vi "AutoCoordinator.vi"(3 "Stop":bool, 4 "Start":bool, 5 "MotionPlanningNotifiers":T1, 6 "Steps":T3[](array[typedef])) -> (1 "Claw Open":bool, 2 "IntakeState":T2)   [LabVIEW 2017]
uses:
  TypeDef/AutoStep.ctl
  TypeDef/AutoWaypointType.ctl
  Pathfinder/Pathfinder-LabVIEW/Pathfinder-Lib/VIs/Waypoint.ctl
  Implements/Arm/TypeDefs/ArmTargetPosition.ctl
  Implements/TypeDefs/IntakeState.ctl
  TypeDefs/RobotComponents/MotionPlanningNotifiers.ctl
  PathPlannerSupport/TypeDefs/DrivePlanRequest.ctl
  PathPlannerSupport/TypeDefs/DrivePlanResponse.ctl
  Pathfinder/Pathfinder-LabVIEW/Pathfinder-Lib/VIs/Segment.ctl
  Implements/Arm/TypeDefs/ArmPlanRequest.ctl
  Implements/Arm/TypeDefs/ArmPlanResponse.ctl
  General/MotionProfiling/TypeDefs/TrajectoryPoint.ctl
  <vilib>/Rock Robotics/WPI/ThirdParty/Phoenix-LabVIEW/Motor Controller/Controls/CTRE_Phoenix_MotorControl_TrajectoryPointTimeDur.ctl
  ArgosLib/Signal Processing/TypeDefs/EdgeDetector_Type.ctl
  ArgosLib/ArgosLib.lvlib
  Pathfinder/Pathfinder-LabVIEW/Pathfinder-Lib/Pathfinder.lvlib
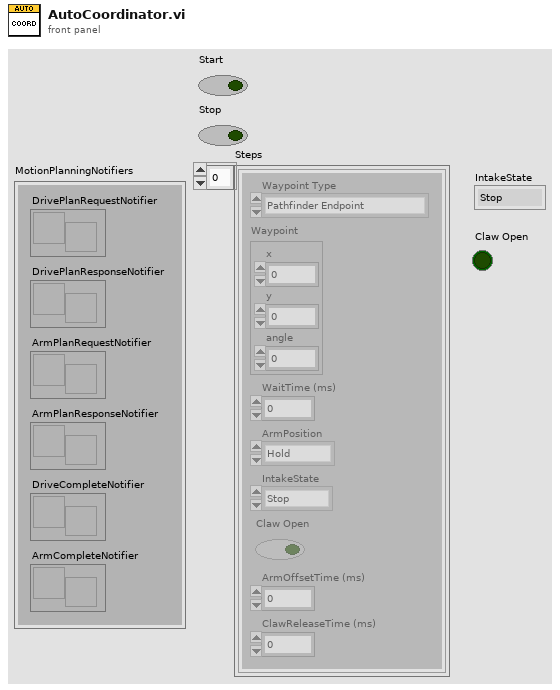
[diagram p1: front panel]
types:
  T1 = typedef "MotionPlanningNotifiers.ctl" = cluster{"DrivePlanRequestNotifier":refnum<notifier>, "DrivePlanResponseNotifier":refnum<notifier>, "ArmPlanRequestNotifier":refnum<notifier>, "ArmPlanResponseNotifier":refnum<notifier>, "DriveCompleteNotifier":refnum<notifier>, "ArmCompleteNotifier":refnum<notifier>}
  T2 = typedef "IntakeState.ctl" = enum16{"Stop", "Forward", "Reverse", "Forward Open"}
  T3 = typedef "AutoStep.ctl" = cluster{"Waypoint Type":T4, "Waypoint":T5, "WaitTime (ms)":u16, "ArmPosition":T6, "IntakeState":T2, "Claw Open":bool, "ArmOffsetTime (ms)":u16, "ClawReleaseTime (ms)":u16}
  T4 = typedef "AutoWaypointType.ctl" = enum16{"Pathfinder Endpoint", "Pathfinder Waypoint", "Zero-Radius Turn Endpoint", "Stationary", "Vision Assist Endpoint", "Stop"}
  T5 = typedef "Pathfinder.lvlib/Waypoint.ctl" = cluster{"x":dbl, "y":dbl, "angle":dbl}
  T6 = typedef "ArmTargetPosition.ctl" = enum16{"Hold", "Switch", "Scale Low", "Scale High", "Climb", "Back Place"}
  T7 = typedef "ArgosLib.lvlib/EdgeDetector_Type.ctl" = enum16{"RisingEdge", "FallingEdge", "Both"}
  T8 = typedef "ArmPlanResponse.ctl" = cluster{"RotateTrajectory":T9[], "ExtendTrajectory":T9[], "PlanTime (ms)":u32, "Execute":bool}
  T9 = typedef "TrajectoryPoint.ctl" = cluster{"Position ":dbl, "Velocity ":dbl, "Time (ms)":T10, "Last Point":bool}
  T10 = typedef "CTRE_Phoenix_MotorControl_TrajectoryPointTimeDur.ctl" = i32
  T11 = typedef "ArmPlanRequest.ctl" = cluster{"Destination":T6, "Preview":bool}
  T12 = typedef "DrivePlanRequest.ctl" = cluster{"Plan Type":T4, "Waypoints":T5[], "Preview":bool}
  T13 = typedef "DrivePlanResponse.ctl" = cluster{"LeftDriveTrajectory":T14[], "RightDriveTrajectory":T14[], "PlanTime (ms)":u32, "Execute":bool}
  T14 = typedef "Pathfinder.lvlib/Segment.ctl" = cluster{"dt":dbl, "x":dbl, "y":dbl, "position":dbl, "velocity":dbl, "acceleration":dbl, "jerk":dbl, "heading":dbl}
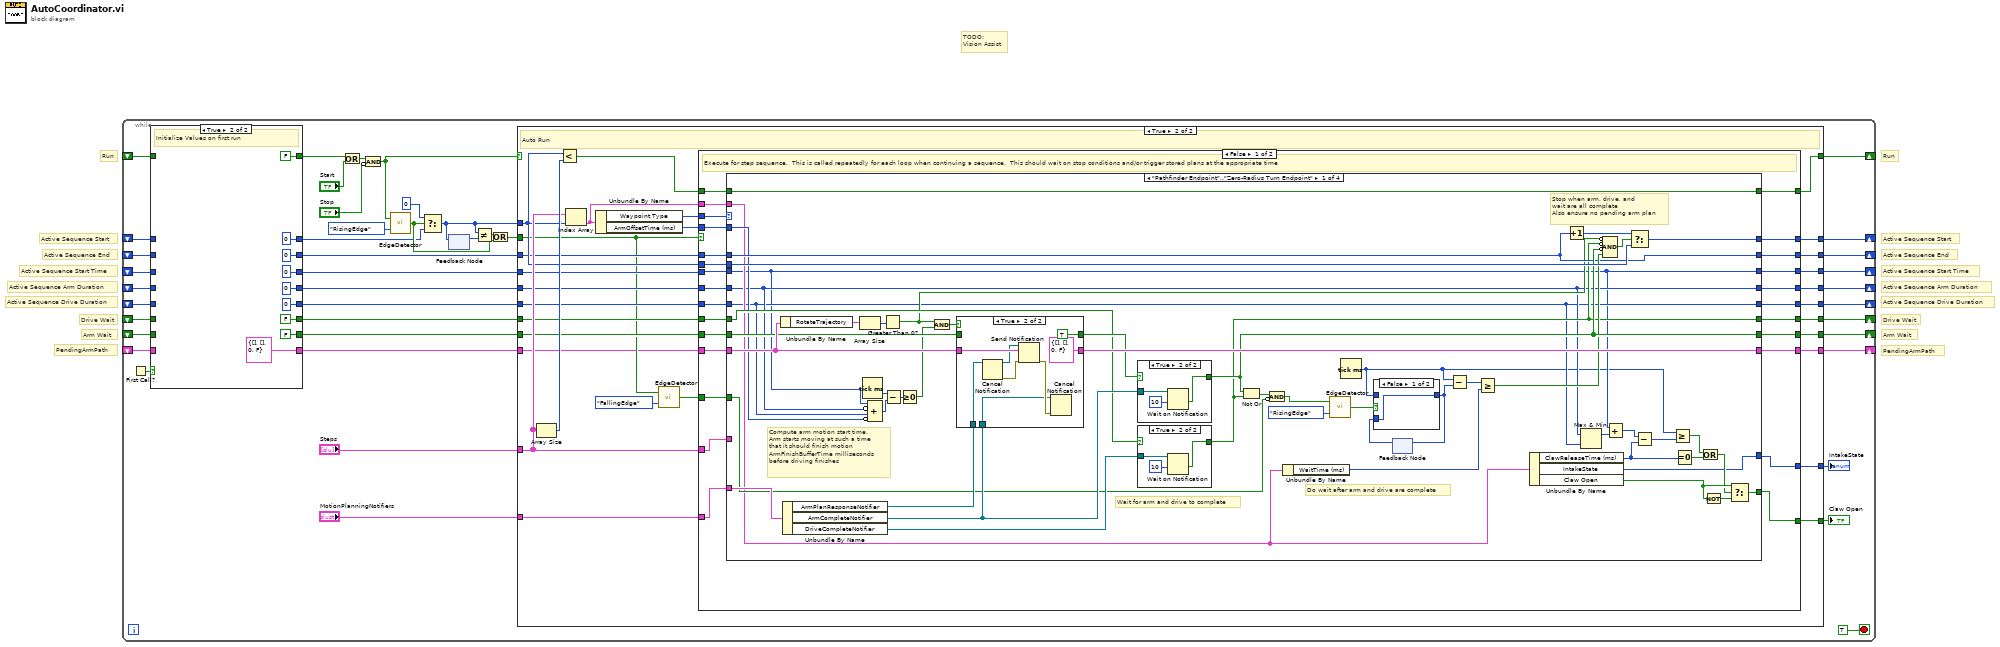
[diagram p0: block diagram]
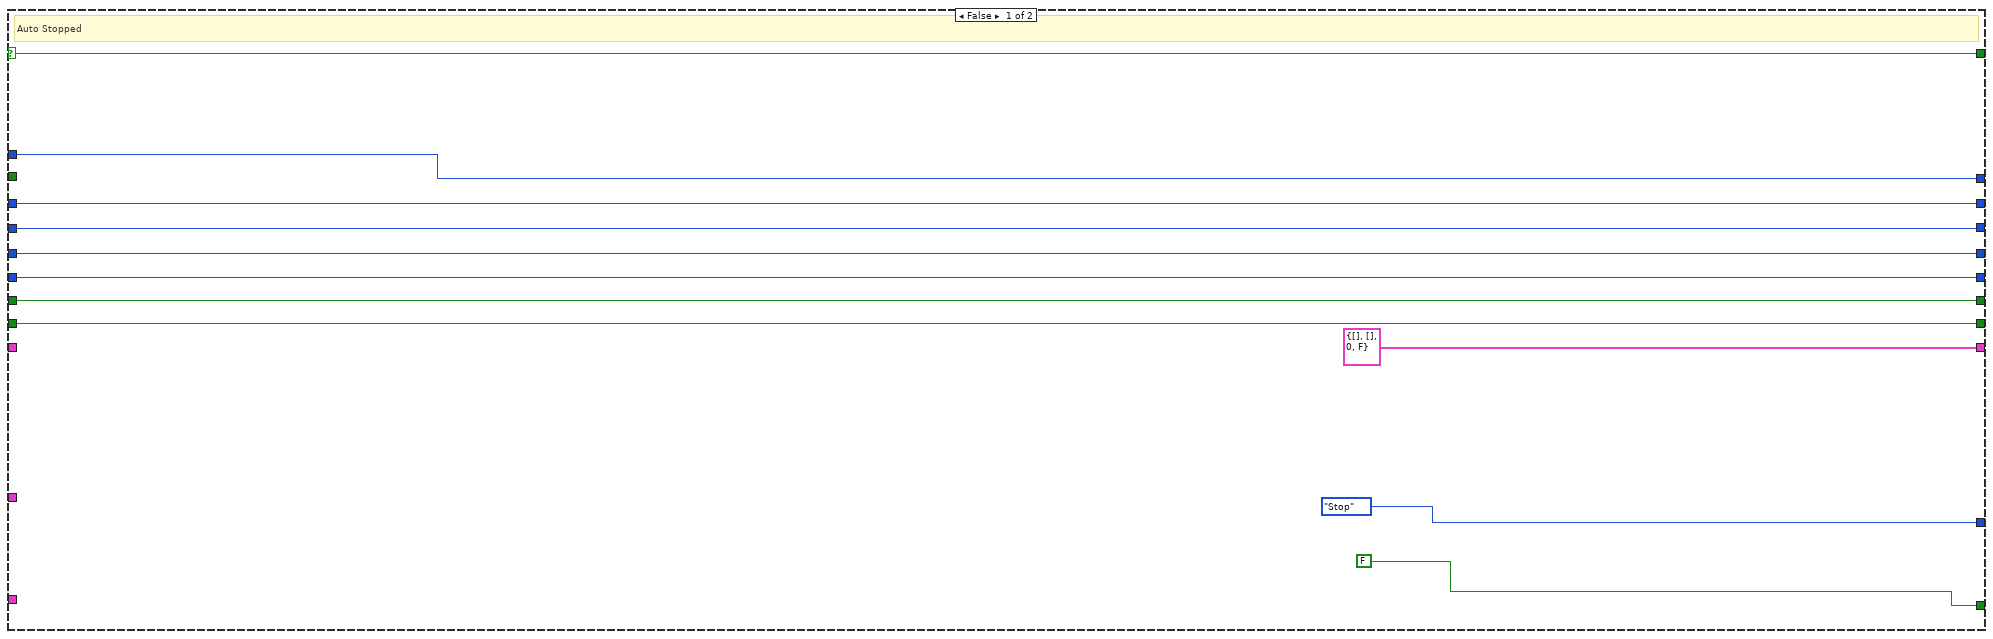
[diagram p3: hidden frame]
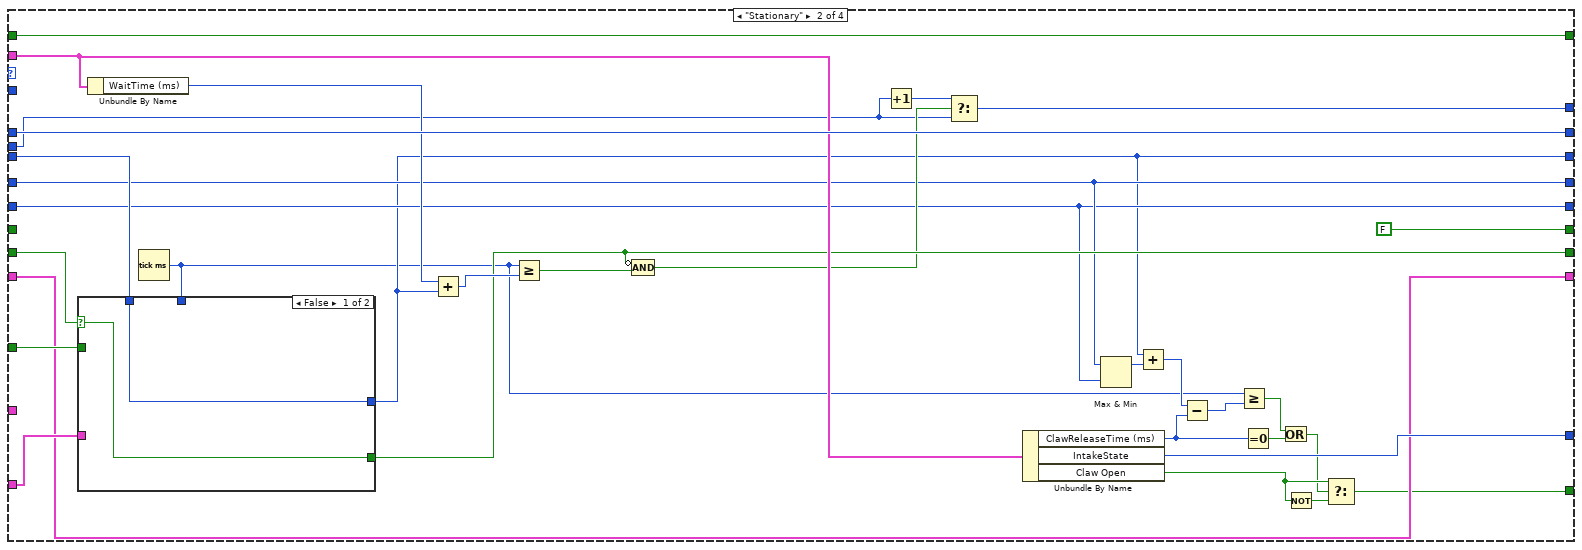
[diagram p8: hidden frame]
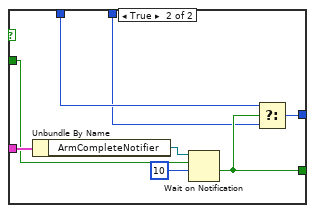
[diagram p9: hidden frame]
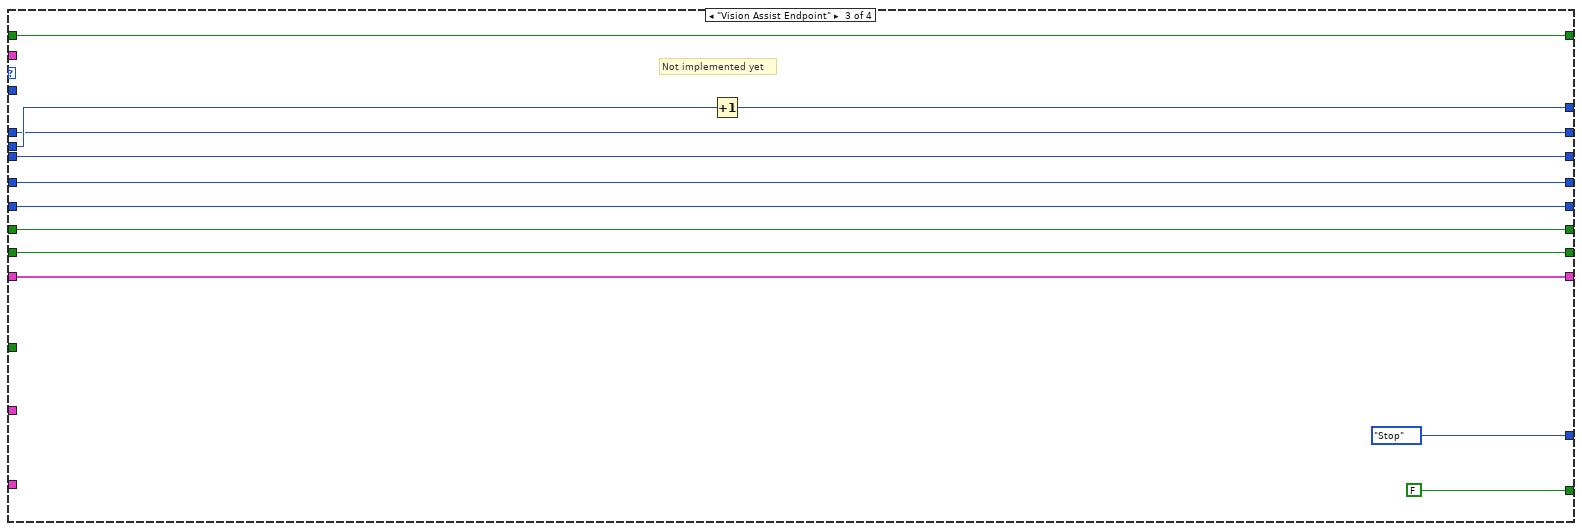
[diagram p10: hidden frame]
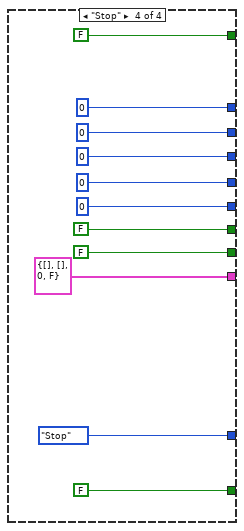
[diagram p11: hidden frame]
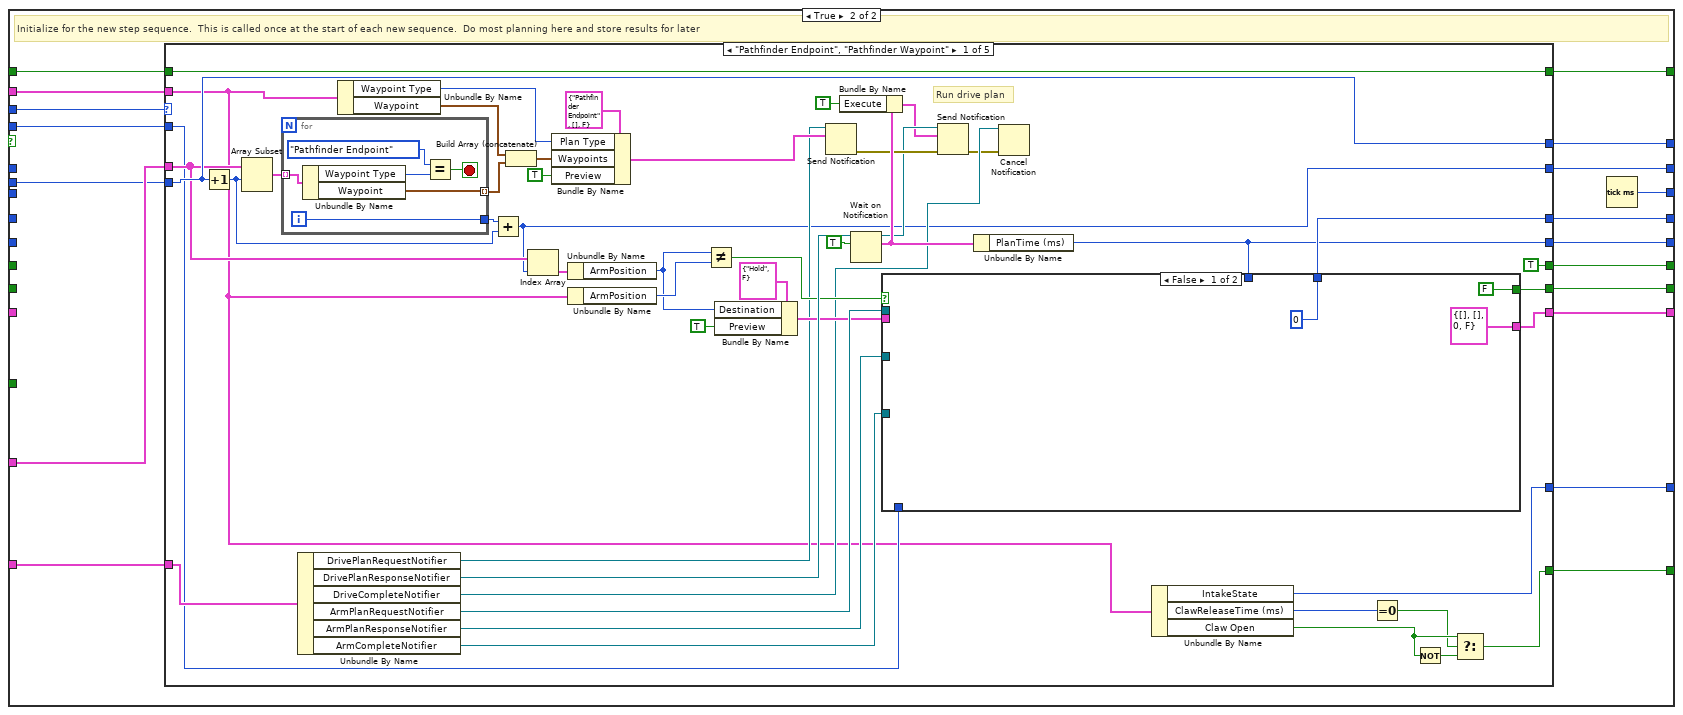
[diagram p12: hidden frame]
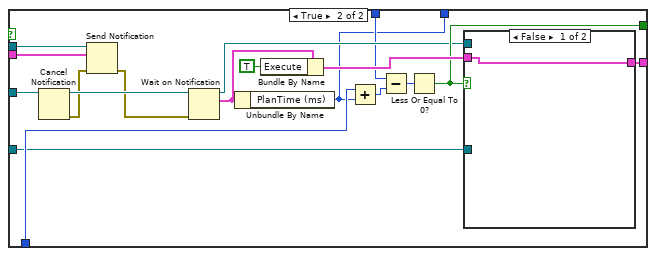
[diagram p13: hidden frame]
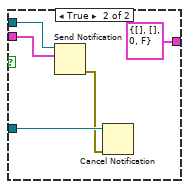
[diagram p14: hidden frame]
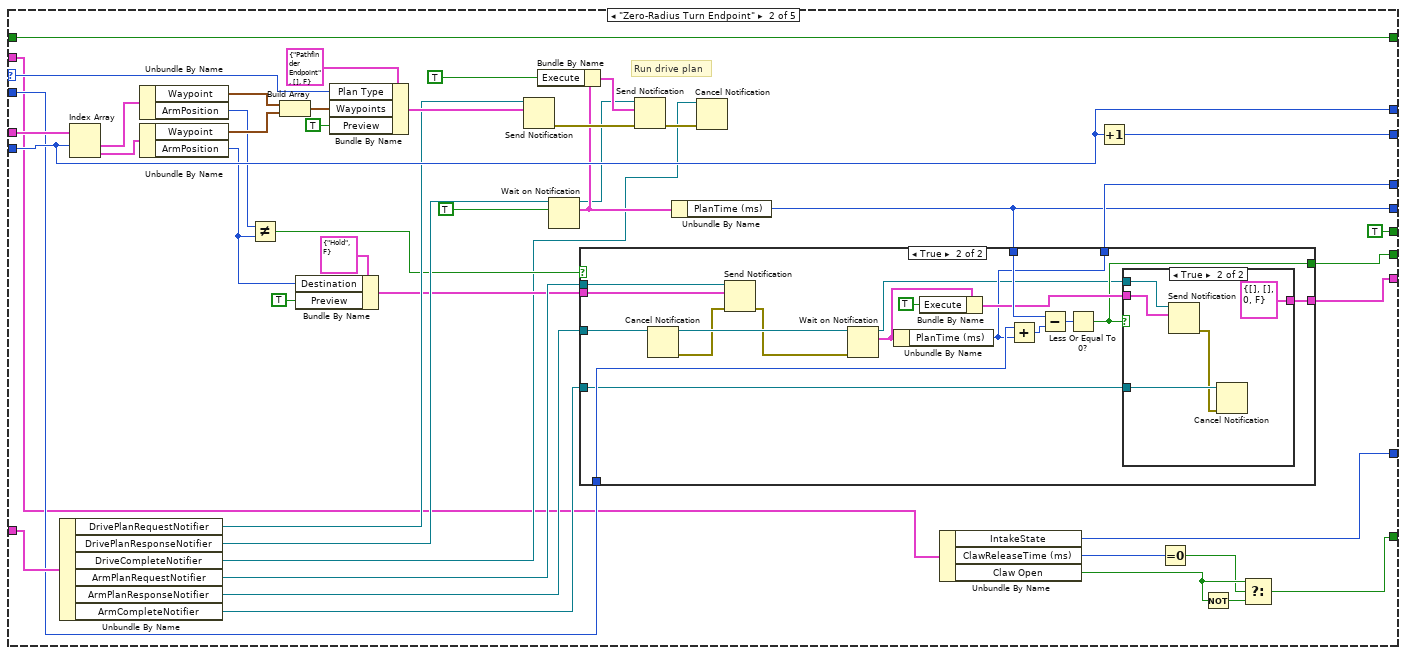
[diagram p15: hidden frame]
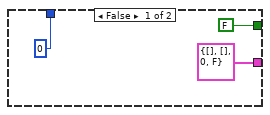
[diagram p16: hidden frame]
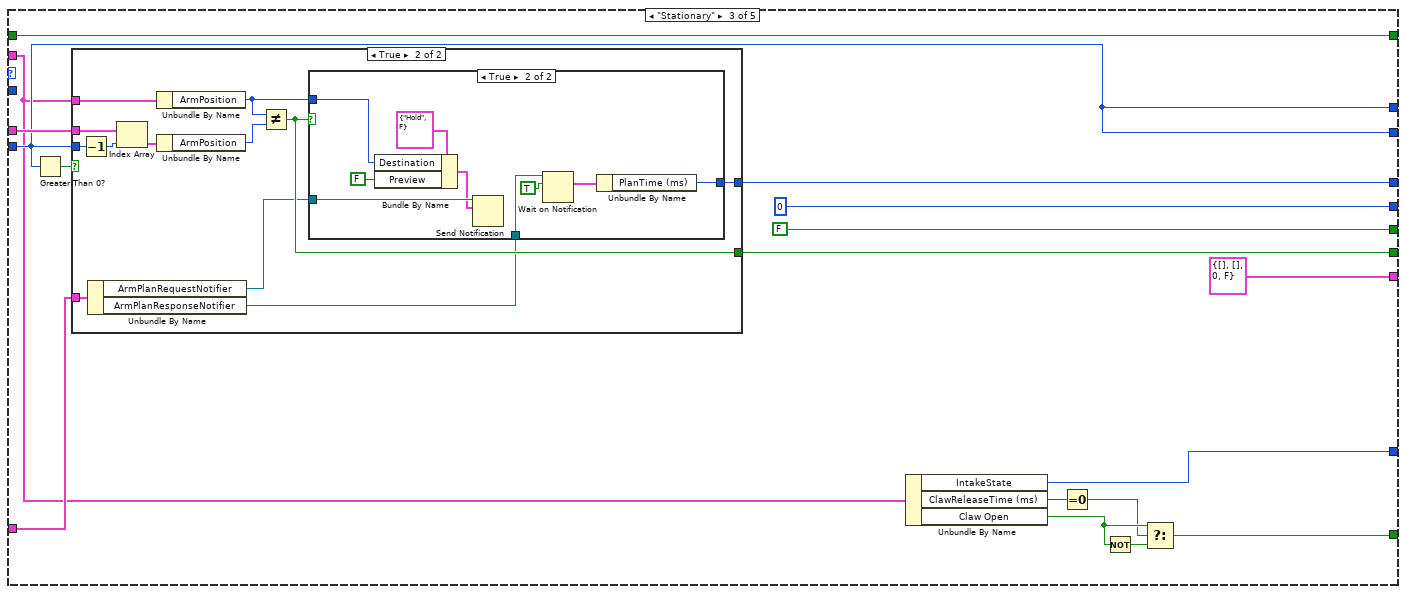
[diagram p18: hidden frame]
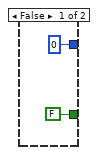
[diagram p19: hidden frame]
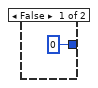
[diagram p20: hidden frame]
diagram:
  # "PendingArmPath"
  # "PendingArmPath"
  # "TODO:\nVision Assist"
  # "Run"
  # "Arm Wait"
  # "Drive Wait"
  # "Active Sequence Drive Duration"
  # "Active Sequence Arm Duration"
  # "Active Sequence Start Time"
  # "Active Sequence End"
  # "Active Sequence Start"
  # "Arm Wait"
  # "Drive Wait"
  # "Active Sequence Drive Duration"
  # "Active Sequence Arm Duration"
  # "Active Sequence Start Time"
  # "Active Sequence End"
  # "Active Sequence Start"
  # "Run"
  n1 = while {
    shift-right: [w37] -> _
    shift-left: _ -> [w17]
    shift-right: [w36] -> _
    shift-left: _ -> [w15]
    shift-right: [w26] -> _
    shift-left: _ -> [w7]
    shift-right: [w25] -> _
    shift-left: _ -> [w6]
    shift-right: [w21] -> _
    shift-left: _ -> [w5]
    shift-right: [w24] -> _
    shift-left: _ -> [w4]
    shift-right: [w23] -> _
    shift-left: _ -> [w3]
    shift-right: [w22] -> _
    shift-left: _ -> [w2]
    shift-right: [w20] -> _
    shift-left: _ -> [w1]
    stop <- TRUE stop-if-true
    n2 = First Call?() -> (First Call?: T/F=w19:bool)
    n3 = case shown="True" w19 {
      tunnel: [w53 FALSE] -> w18
      tunnel: w17 -> [w53 _]
      tunnel: [w52 0] -> w16
      tunnel: w15 -> [w52 _]
      tunnel: [w51 0] -> w14
      tunnel: [w50 u32 0 ("millisecond timer value")] -> w13
      tunnel: [w49 u32 0 ("PlanTime (ms)")] -> w12
      tunnel: [w48 u32 0 ("PlanTime (ms)")] -> w11
      tunnel: [w47 FALSE ("timed out?")] -> w10
      tunnel: [w46 FALSE ("timed out?")] -> w9
      tunnel: [w45 T8 {"RotateTrajectory"=[], "ExtendTrajectory"=[], "PlanTime (ms)"=0, "Execute"=FALSE} ("ArmPlanResponse")] -> w8
      tunnel: w7 -> [w51 _]
      tunnel: w6 -> [w50 _]
      tunnel: w5 -> [w49 _]
      tunnel: w4 -> [w48 _]
      tunnel: w3 -> [w47 _]
      tunnel: w2 -> [w46 _]
      tunnel: w1 -> [w45 _]
      frame False {
      }
      frame True {
        # "Initialize Values on first run"
      }
    }
    n4 = Or(x=w18, y="Start") -> (x .or. y?=w42:bool)
    n5 = Compound Arithmetic op=AND(w42, invert "Stop") -> (w38:bool)
    n6 = call "EdgeDetector.vi"("DetectorType"=EdgeDetector_Type."RisingEdge", "Input"=w38) -> ("Edge"=w28:bool)
    n7 = Select(t=0, s=w28, f=w16) -> (s? t:f=w30:i32)
    n8 = feedback-in #1(w30) -> ()
    n9 = feedback #1() -> (w31:i32)  [unwired: 1 in]
    n10 = Not Equal?(x=w30, y=w31) -> (x != y?=w29:bool)
    n11 = Or(x=w29, y=w28) -> (x .or. y?=w27:bool)
    n12 = case shown="True" w38 {
      selector: w38 -> [w72 _]
      tunnel: [w72 w75] -> w37
      tunnel: w30 -> [w73 w100]
      tunnel: [w73 w99] -> w36
      tunnel: "Steps" -> [_ w101]
      tunnel: [IntakeState."Stop" ("IntakeState") w94] -> w34
      tunnel: [FALSE ("Claw Open") w93] -> w33
      tunnel: "MotionPlanningNotifiers" -> [_ w90]
      tunnel: w27 -> [_ w81]
      tunnel: [w69 w98] -> w26
      tunnel: [w68 w97] -> w25
      tunnel: w13 -> [w68 w96]
      tunnel: [w66 w95] -> w24
      tunnel: [w65 w92] -> w23
      tunnel: [w64 w91] -> w22
      tunnel: [w67 w89] -> w21
      tunnel: w14 -> [w69 w82]
      tunnel: w12 -> [w67 w83]
      tunnel: w11 -> [w66 w84]
      tunnel: w10 -> [w65 w86]
      tunnel: w9 -> [w64 w85]
      tunnel: [T8 {"RotateTrajectory"=[], "ExtendTrajectory"=[], "PlanTime (ms)"=0, "Execute"=FALSE} ("ArmPlanResponse") w78] -> w20
      tunnel: w8 -> [_ w77]
      frame False {
        # "Auto Stopped"
      }
      frame True {
        # "Auto Run"
        n13 = Array Size(array=w101) -> (size(s)=w102:i32)
        n14 = Less?(x=w100, y=w102) -> (x < y?=w76:bool)
        n15 = Index Array(array=w101, index=w100) -> (element=w87:T3)
        n16 = Unbundle By Name(w87) -> ("Waypoint Type"=w88:T4, "ArmOffsetTime (ms)"=w74:u16)
        n17 = call "EdgeDetector.vi"("DetectorType"=EdgeDetector_Type."FallingEdge", "Input"=w81) -> ("Edge"=w79:bool)
        n18 = case shown="False" w81 {
          tunnel: w101 -> [w125 w283]
          tunnel: w100 -> [w119 w282]
          tunnel: [w118 w281] -> w99
          tunnel: [w117 w280] -> w98
          tunnel: [w108 w279] -> w97
          tunnel: w96 -> [w109 _]
          tunnel: [w115 w278] -> w95
          tunnel: [w112 w277] -> w94
          tunnel: [w111 w276] -> w93
          tunnel: [w114 w275] -> w92
          tunnel: [w113 w274] -> w91
          tunnel: w90 -> [w124 w273]
          tunnel: [w116 w272] -> w89
          tunnel: w88 -> [w128 w271]
          tunnel: w87 -> [w126 w270]
          tunnel: w86 -> [w123 _]
          tunnel: w85 -> [w122 _]
          tunnel: w84 -> [w121 _]
          tunnel: w83 -> [w120 _]
          tunnel: w82 -> [w127 _]
          tunnel: w79 -> [w110 _]
          tunnel: [w107 w269] -> w78
          tunnel: w77 -> [w106 _]
          tunnel: w76 -> [w105 w268]
          tunnel: [w104 w267] -> w75
          tunnel: w74 -> [w103 w266]
          frame False {
            # "Execute for step sequence.  This is called repeatedly for each loop when continuing a sequence.  This should wait on stop conditions and/or trigger stored plans at the appropriate time"
            n19 = case shown="\"Pathfinder Endpoint\"..\"Zero-Radius Turn Endpoint\"" w128 {
              tunnel: w127 -> [w151 w227 w248 _]
              tunnel: w126 -> [w133 w226 _ _]
              tunnel: w125 -> [_ _ _ _]
              tunnel: w124 -> [w174 w230 _ _]
              tunnel: w123 -> [w150 _ w252 _]
              tunnel: w122 -> [w170 w232 w251 _]
              tunnel: w121 -> [w131 w208 w253 _]
              tunnel: w120 -> [w132 w209 w254 _]
              tunnel: w109 -> [w130 w225 w245 _]
              tunnel: w119 -> [w178 w217 w250 _]
              tunnel: [w180 w222 w249 0] -> w118
              tunnel: [w151 w227 w248 0] -> w117
              tunnel: [w132 w209 w254 u32 0 ("PlanTime (ms)")] -> w116
              tunnel: [w131 w208 w253 u32 0 ("PlanTime (ms)")] -> w115
              tunnel: [w148 FALSE w252 FALSE ("timed out?")] -> w114
              tunnel: [w162 w220 w251 FALSE ("timed out?")] -> w113
              tunnel: [w134 w231 IntakeState."Stop" ("IntakeState") IntakeState."Stop" ("IntakeState")] -> w112
              tunnel: [w135 w214 FALSE ("Claw Open") FALSE ("Claw Open")] -> w111
              tunnel: w110 -> [w160 w229 _ _]
              tunnel: [w130 w203 w245 u32 0 ("millisecond timer value")] -> w108
              tunnel: [w171 w216 w244 T8 {"RotateTrajectory"=[], "ExtendTrajectory"=[], "PlanTime (ms)"=0, "Execute"=FALSE} ("ArmPlanResponse")] -> w107
              tunnel: w106 -> [w172 w216 w244 _]
              tunnel: w105 -> [w146 w215 w243 _]
              tunnel: [w146 w215 w243 FALSE] -> w104
              tunnel: w103 -> [w145 _ _ _]
              frame "Pathfinder Endpoint".."Zero-Radius Turn Endpoint" {
                # "Do wait after arm and drive are complete"
                # "Wait for arm and drive to complete"
                # "Stop when arm, drive, and\nwait are all complete\nAlso ensure no pending arm plan"
                # "Compute arm motion start time.\nArm starts moving at such a time\nthat it should finish motion\nArmFinishBufferTime milliseconds\nbefore driving finishes"
                n20 = Unbundle By Name(w172) -> ("RotateTrajectory"=w177:T9[])
                n21 = Unbundle By Name(w174) -> ("ArmPlanResponseNotifier"=w173:refnum<notifier>, "ArmCompleteNotifier"=w164:refnum<notifier>, "DriveCompleteNotifier"=w165:refnum<notifier>)
                n22 = Array Size(array=w177) -> (size(s)=w176:i32)
                n23 = Tick Count (ms)() -> (millisecond timer value=w175:u32)
                n24 = Compound Arithmetic op=ADD(w130, invert w132, w131, invert w145) -> (w147:u32)
                n25 = Greater Than 0?(x=w176) -> (x > 0?=w149:bool)
                n26 = Subtract(x=w175, y=w147) -> (x-y=w168:i32)
                n27 = Greater Or Equal To 0?(x=w168) -> (x >= 0?=w167:bool)
                n28 = And(x=w149, y=w167) -> (x .and. y?=w169:bool)
                n29 = case shown="True" w169 {
                  tunnel: [w191 TRUE] -> w163
                  tunnel: w173 -> [_ w195]
                  tunnel: w172 -> [w192 w198]
                  tunnel: w164 -> [_ w197]
                  tunnel: [w192 T8 {"RotateTrajectory"=[], "ExtendTrajectory"=[], "PlanTime (ms)"=0, "Execute"=FALSE} ("ArmPlanResponse")] -> w171
                  tunnel: w170 -> [w191 _]
                  frame False {
                  }
                  frame True {
                    n30 = Cancel Notification(0:w195) -> (8:w194:refnum<notifier>, 11:w193:errorcluster)  [unwired: 1 in, 1 out]
                    n31 = Send Notification(notification=w198, notifier=w194, error in (no error)=w193) -> (error out=w199:errorcluster)  [unwired: 1 out]
                    n32 = Cancel Notification(0:w197, 3:w199) -> ()  [unwired: 3 out]
                  }
                }
                n33 = case shown="True" w163 {
                  selector: w163 -> [w187 _]
                  tunnel: w164 -> [_ w189]
                  tunnel: [w187 w188] -> w162
                  frame False {
                  }
                  frame True {
                    n34 = Wait on Notification(notifier=w189, timeout in ms (-1)=10) -> (timed out?=w188:bool)  [unwired: 2 in, 3 out]
                  }
                }
                n35 = case shown="True" w150 {
                  selector: w150 -> [w183 _]
                  tunnel: w165 -> [_ w185]
                  tunnel: [w183 w184] -> w148
                  frame False {
                  }
                  frame True {
                    n36 = Wait on Notification(notifier=w185, timeout in ms (-1)=10) -> (timed out?=w184:bool)  [unwired: 2 in, 3 out]
                  }
                }
                n37 = Not Or(1:w148, 2:w162) -> (0:w161:bool)
                n38 = Compound Arithmetic op=AND(w161, invert w160) -> (w158:bool)
                n39 = Unbundle By Name(w133) -> ("WaitTime (ms)"=w153:u16)
                n40 = call "EdgeDetector.vi"("DetectorType"=EdgeDetector_Type."RisingEdge", "Input"=w158) -> ("Edge"=w157:bool)
                n41 = Tick Count (ms)() -> (millisecond timer value=w129:u32)
                n42 = feedback #2() -> (w156:u32)  [unwired: 1 in]
                n43 = case shown="False" w157 {
                  tunnel: w129 -> [_ w182]
                  tunnel: [w181 w182] -> w155
                  tunnel: w156 -> [w181 _]
                  frame False {
                  }
                  frame True {
                  }
                }
                n44 = feedback-in #2(w155) -> ()
                n45 = Subtract(x=w129, y=w155) -> (x-y=w154:u32)
                n46 = Greater Or Equal?(x=w154, y=w153) -> (x >= y?=w152:bool)
                n47 = Unbundle By Name(w133) -> ("ClawReleaseTime (ms)"=w140:u16, "IntakeState"=w134:T2, "Claw Open"=w143:bool)
                n48 = Increment(x=w151) -> (x+1=w179:i32)
                n49 = Max & Min(x=w132, y=w131) -> (max(x,y)=w137:u32)  [unwired: 1 out]
                n50 = Compound Arithmetic op=AND(invert w149, invert w148, invert w162, w152) -> (w166:bool)
                n51 = Add(x=w130, y=w137) -> (x+y=w138:u32)
                n52 = Select(t=w179, s=w166, f=w178) -> (s? t:f=w180:i32)
                n53 = Subtract(x=w138, y=w140) -> (x-y=w136:u32)
                n54 = Greater Or Equal?(x=w129, y=w136) -> (x >= y?=w139:bool)
                n55 = Equal To 0?(x=w140) -> (x = 0?=w142:bool)
                n56 = Or(x=w139, y=w142) -> (x .or. y?=w141:bool)
                n57 = Not(x=w143) -> (.not. x?=w144:bool)
                n58 = Select(t=w143, s=w141, f=w144) -> (s? t:f=w135:bool)
              }
              frame "Stationary" {
                n59 = Unbundle By Name(w226) -> ("WaitTime (ms)"=w223:u16)
                n60 = Tick Count (ms)() -> (millisecond timer value=w201:u32)
                n61 = case shown="False" w232 {
                  selector: w232 -> [w234 _]
                  tunnel: w230 -> [_ w242]
                  tunnel: w229 -> [_ w239]
                  tunnel: [w234 w238] -> w220
                  tunnel: w225 -> [w233 w237]
                  tunnel: w201 -> [_ w236]
                  tunnel: [w233 w235] -> w203
                  frame False {
                  }
                  frame True {
                    n62 = Unbundle By Name(w242) -> ("ArmCompleteNotifier"=w241:refnum<notifier>)
                    n63 = Wait on Notification(notifier=w241, ignore previous (F)=w239, timeout in ms (-1)=10) -> (timed out?=w238:bool)  [unwired: 1 in, 3 out]
                    n64 = Select(t=w237, s=w238, f=w236) -> (s? t:f=w235:u32)
                  }
                }
                n65 = Add(x=w223, y=w203) -> (x+y=w224:u32)
                n66 = Greater Or Equal?(x=w201, y=w224) -> (x >= y?=w221:bool)
                n67 = Compound Arithmetic op=AND(invert w220, w221) -> (w219:bool)
                n68 = Increment(x=w217) -> (x+1=w218:i32)
                n69 = Select(t=w218, s=w219, f=w217) -> (s? t:f=w222:i32)
                n70 = Unbundle By Name(w226) -> ("ClawReleaseTime (ms)"=w207:u16, "IntakeState"=w231:T2, "Claw Open"=w212:bool)
                n71 = Max & Min(x=w209, y=w208) -> (max(x,y)=w204:u32)  [unwired: 1 out]
                n72 = Add(x=w203, y=w204) -> (x+y=w205:u32)
                n73 = Subtract(x=w205, y=w207) -> (x-y=w202:u32)
                n74 = Greater Or Equal?(x=w201, y=w202) -> (x >= y?=w206:bool)
                n75 = Equal To 0?(x=w207) -> (x = 0?=w211:bool)
                n76 = Or(x=w206, y=w211) -> (x .or. y?=w210:bool)
                n77 = Not(x=w212) -> (.not. x?=w213:bool)
                n78 = Select(t=w212, s=w210, f=w213) -> (s? t:f=w214:bool)
              }
              frame "Vision Assist Endpoint" {
                # "Not implemented yet"
                n79 = Increment(x=w250) -> (x+1=w249:i32)
              }
              frame "Stop" {
              }
            }
          }
          frame True {
            # "Initialize for the new step sequence.  This is called once at the start of each new sequence.  Do most planning here and store results for later"
            n80 = case shown="\"Pathfinder Endpoint\", \"Pathfinder Waypoint\"" w271 {
              selector: w271 -> [_ w405 _ _ _]
              tunnel: w283 -> [w300 w410 w451 _ _]
              tunnel: w282 -> [w301 w408 w447 w488 _]
              tunnel: w270 -> [w288 w368 w440 _ _]
              tunnel: [w301 w408 w447 w484 0] -> w281
              tunnel: [w299 w409 w447 w484 0] -> w280
              tunnel: [w302 w377 u16 0 u32 0 ("PlanTime (ms)") u32 0 ("PlanTime (ms)")] -> w278
              tunnel: [w284 w365 w439 IntakeState."Stop" ("IntakeState") IntakeState."Stop" ("IntakeState")] -> w277
              tunnel: [w287 w367 w438 FALSE ("Claw Open") FALSE ("Claw Open")] -> w276
              tunnel: [TRUE TRUE FALSE FALSE FALSE] -> w275
              tunnel: [w294 w375 w450 FALSE FALSE] -> w274
              tunnel: w273 -> [w304 w399 w449 _ _]
              tunnel: [w303 w379 w448 u32 0 ("PlanTime (ms)") u32 0 ("PlanTime (ms)")] -> w272
              tunnel: [w295 w380 T8 {"RotateTrajectory"=[], "ExtendTrajectory"=[], "PlanTime (ms)"=0, "Execute"=FALSE} ("ArmPlanResponse") T8 {"RotateTrajectory"=[], "ExtendTrajectory"=[], "PlanTime (ms)"=0, "Execute"=FALSE} ("ArmPlanResponse") T8 {"RotateTrajectory"=[], "ExtendTrajectory"=[], "PlanTime (ms)"=0, "Execute"=FALSE} ("ArmPlanResponse")] -> w269
              tunnel: w268 -> [w292 w373 w445 w479 _]
              tunnel: [w292 w373 w445 w479 FALSE] -> w267
              tunnel: w266 -> [w291 w372 _ _ _]
              frame "Pathfinder Endpoint", "Pathfinder Waypoint" {
                # "Run drive plan"
                n81 = Increment(x=w301) -> (x+1=w329:i32)
                n82 = Array Subset(array=w300, index=w329) -> (w331:T3[])  [unwired: 1 in]
                n83 = for {
                  tunnel: w331 -> [w364] mode=indexing
                  tunnel: [w360] -> w330
                  tunnel: [w359] -> w325 mode=indexing
                  i -> [w360]
                  stop <- w361 stop-if-true
                  n84 = Unbundle By Name(w364) -> ("Waypoint Type"=w363:T4, "Waypoint"=w359:T5)
                  n85 = Equal?(x=AutoWaypointType."Pathfinder Endpoint", y=w363) -> (x = y?=w361:bool)
                }
                n86 = Unbundle By Name(w304) -> ("DrivePlanRequestNotifier"=w305:refnum<notifier>, "DrivePlanResponseNotifier"=w322:refnum<notifier>, "DriveCompleteNotifier"=w312:refnum<notifier>, "ArmPlanRequestNotifier"=w317:refnum<notifier>, "ArmPlanResponseNotifier"=w313:refnum<notifier>, "ArmCompleteNotifier"=w311:refnum<notifier>)
                n87 = Unbundle By Name(w288) -> ("Waypoint Type"=w327:T4, "Waypoint"=w326:T5)
                n88 = Add(x=w330, y=w329) -> (x+y=w299:i32)
                n89 = Build Array (concatenate)(w326, w325) -> (w324:T5[])
                n90 = Index Array(array=w300, index=w299) -> (element=w298:T3)
                n91 = Bundle By Name(cluster=T12 {"Plan Type"=enum."Pathfinder Endpoint", "Waypoints"=[], "Preview"=FALSE} ("DrivePlanRequest"), "Plan Type"=w327, "Waypoints"=w324, "Preview"=TRUE) -> (w306:T12)
                n92 = Unbundle By Name(w298) -> ("ArmPosition"=w296:T6)
                n93 = Unbundle By Name(w288) -> ("ArmPosition"=w297:T6)
                n94 = Not Equal?(x=w296, y=w297) -> (x != y?=w314:bool)
                n95 = Bundle By Name(cluster=T11 {"Destination"=enum."Hold", "Preview"=FALSE} ("ArmPlanRequest"), "Destination"=w296, "Preview"=TRUE) -> (w316:T11)
                n96 = Send Notification(notification=w306, notifier=w305) -> (error out=w309:errorcluster)  [unwired: 1 in, 1 out]
                n97 = Wait on Notification(notifier=w322, ignore previous (F)=TRUE) -> (notifier out=w308:refnum<notifier>, notification=w320:T13)  [unwired: 2 in, 2 out]
                n98 = Bundle By Name(cluster=w320, "Execute"=TRUE) -> (w307:T13)
                n99 = Send Notification(notification=w307, notifier=w308, error in (no error)=w309) -> (error out=w310:errorcluster)  [unwired: 1 out]
                n100 = Unbundle By Name(w320) -> ("PlanTime (ms)"=w302:u32)
                n101 = case shown="False" w314 {
                  tunnel: w317 -> [_ w352]
                  tunnel: w316 -> [_ w351]
                  tunnel: w313 -> [_ w340]
                  tunnel: [T8 {"RotateTrajectory"=[], "ExtendTrajectory"=[], "PlanTime (ms)"=0, "Execute"=FALSE} ("ArmPlanResponse") w343] -> w295
                  tunnel: [u32 0 ("PlanTime (ms)") w335] -> w303
                  tunnel: w311 -> [_ w341]
                  tunnel: w291 -> [_ w350]
                  tunnel: w302 -> [_ w336]
                  tunnel: [FALSE w344] -> w294
                  frame False {
                  }
                  frame True {
                    n102 = Cancel Notification(0:w340) -> (8:w339:refnum<notifier>, 11:w338:errorcluster)  [unwired: 1 in, 1 out]
                    n103 = Send Notification(notification=w351, notifier=w352, error in (no error)=w338) -> (error out=w337:errorcluster)  [unwired: 1 out]
                    n104 = Wait on Notification(notifier=w339, error in (no error)=w337) -> (notifier out=w342:refnum<notifier>, notification=w347:T8)  [unwired: 2 in, 2 out]
                    n105 = Unbundle By Name(w347) -> ("PlanTime (ms)"=w335:u32)
                    n106 = Bundle By Name(cluster=w347, "Execute"=TRUE) -> (w345:T8)
                    n107 = Add(x=w350, y=w335) -> (x+y=w349:u32)
                    n108 = Subtract(x=w336, y=w349) -> (x-y=w348:i32)
                    n109 = Less Or Equal To 0?(x=w348) -> (x <= 0?=w344:bool)
                    n110 = case shown="False" w344 {
                      tunnel: w345 -> [w353 w357]
                      tunnel: [w353 T8 {"RotateTrajectory"=[], "ExtendTrajectory"=[], "PlanTime (ms)"=0, "Execute"=FALSE} ("ArmPlanResponse")] -> w343
                      tunnel: w342 -> [_ w358]
                      tunnel: w341 -> [_ w356]
                      frame False {
                      }
                      frame True {
                        n111 = Send Notification(notification=w357, notifier=w358) -> (error out=w354:errorcluster)  [unwired: 1 in, 1 out]
                        n112 = Cancel Notification(0:w356, 3:w354) -> ()  [unwired: 3 out]
                      }
                    }
                  }
                }
                n113 = Cancel Notification(0:w312, 3:w310) -> ()  [unwired: 3 out]
                n114 = Unbundle By Name(w288) -> ("IntakeState"=w284:T2, "ClawReleaseTime (ms)"=w285:u16, "Claw Open"=w289:bool)
                n115 = Equal To 0?(x=w285) -> (x = 0?=w286:bool)
                n116 = Not(x=w289) -> (.not. x?=w290:bool)
                n117 = Select(t=w289, s=w286, f=w290) -> (s? t:f=w287:bool)
              }
              frame "Zero-Radius Turn Endpoint" {
                # "Run drive plan"
                n118 = Unbundle By Name(w399) -> ("DrivePlanRequestNotifier"=w392:refnum<notifier>, "DrivePlanResponseNotifier"=w397:refnum<notifier>, "DriveCompleteNotifier"=w381:refnum<notifier>, "ArmPlanRequestNotifier"=w388:refnum<notifier>, "ArmPlanResponseNotifier"=w383:refnum<notifier>, "ArmCompleteNotifier"=w378:refnum<notifier>)
                n119 = Index Array(array=w410, index #1=w408) -> (element #1=w407:T3, element #2=w374:T3)  [unwired: 1 in]
                n120 = Unbundle By Name(w407) -> ("Waypoint"=w404:T5, "ArmPosition"=w390:T6)
                n121 = Unbundle By Name(w374) -> ("Waypoint"=w403:T5, "ArmPosition"=w386:T6)
                n122 = Not Equal?(x=w390, y=w386) -> (x != y?=w384:bool)
                n123 = Build Array(w404, w403) -> (w402:T5[])
                n124 = Bundle By Name(cluster=T11 {"Destination"=enum."Hold", "Preview"=FALSE} ("ArmPlanRequest"), "Destination"=w386, "Preview"=TRUE) -> (w387:T11)
                n125 = Bundle By Name(cluster=T12 {"Plan Type"=enum."Pathfinder Endpoint", "Waypoints"=[], "Preview"=FALSE} ("DrivePlanRequest"), "Plan Type"=w405, "Waypoints"=w402, "Preview"=TRUE) -> (w401:T12)
                n126 = Send Notification(notification=w401, notifier=w392) -> (error out=w398:errorcluster)  [unwired: 1 in, 1 out]
                n127 = Wait on Notification(notifier=w397, ignore previous (F)=TRUE) -> (notifier out=w391:refnum<notifier>, notification=w395:T13)  [unwired: 2 in, 2 out]
                n128 = Bundle By Name(cluster=w395, "Execute"=TRUE) -> (w393:T13)
                n129 = Send Notification(notification=w393, notifier=w391, error in (no error)=w398) -> (error out=w382:errorcluster)  [unwired: 1 out]
                n130 = Unbundle By Name(w395) -> ("PlanTime (ms)"=w377:u32)
                n131 = case shown="True" w384 {
                  tunnel: w388 -> [_ w431]
                  tunnel: w387 -> [_ w430]
                  tunnel: w383 -> [_ w429]
                  tunnel: [T8 {"RotateTrajectory"=[], "ExtendTrajectory"=[], "PlanTime (ms)"=0, "Execute"=FALSE} ("ArmPlanResponse") w419] -> w380
                  tunnel: [u32 0 ("PlanTime (ms)") w421] -> w379
                  tunnel: w378 -> [_ w417]
                  tunnel: w372 -> [_ w428]
                  tunnel: w377 -> [_ w426]
                  tunnel: [FALSE w420] -> w375
                  frame False {
                  }
                  frame True {
                    n132 = Cancel Notification(0:w429) -> (8:w416:refnum<notifier>, 11:w415:errorcluster)  [unwired: 1 in, 1 out]
                    n133 = Send Notification(notification=w430, notifier=w431, error in (no error)=w415) -> (error out=w414:errorcluster)  [unwired: 1 out]
                    n134 = Wait on Notification(notifier=w416, error in (no error)=w414) -> (notifier out=w418:refnum<notifier>, notification=w424:T8)  [unwired: 2 in, 2 out]
                    n135 = Unbundle By Name(w424) -> ("PlanTime (ms)"=w421:u32)
                    n136 = Bundle By Name(cluster=w424, "Execute"=TRUE) -> (w422:T8)
                    n137 = Add(x=w428, y=w421) -> (x+y=w427:u32)
                    n138 = Subtract(x=w426, y=w427) -> (x-y=w425:i32)
                    n139 = Less Or Equal To 0?(x=w425) -> (x <= 0?=w420:bool)
                    n140 = case shown="True" w420 {
                      tunnel: w422 -> [w432 w436]
                      tunnel: [w432 T8 {"RotateTrajectory"=[], "ExtendTrajectory"=[], "PlanTime (ms)"=0, "Execute"=FALSE} ("ArmPlanResponse")] -> w419
                      tunnel: w418 -> [_ w437]
                      tunnel: w417 -> [_ w435]
                      frame False {
                      }
                      frame True {
                        n141 = Send Notification(notification=w436, notifier=w437) -> (error out=w433:errorcluster)  [unwired: 1 in, 1 out]
                        n142 = Cancel Notification(0:w435, 3:w433) -> ()  [unwired: 3 out]
                      }
                    }
                  }
                }
                n143 = Cancel Notification(0:w381, 3:w382) -> ()  [unwired: 3 out]
                n144 = Unbundle By Name(w368) -> ("IntakeState"=w365:T2, "ClawReleaseTime (ms)"=w366:u16, "Claw Open"=w370:bool)
                n145 = Increment(x=w408) -> (x+1=w409:i32)
                n146 = Equal To 0?(x=w366) -> (x = 0?=w369:bool)
                n147 = Not(x=w370) -> (.not. x?=w371:bool)
                n148 = Select(t=w370, s=w369, f=w371) -> (s? t:f=w367:bool)
              }
              frame "Stationary" {
                n149 = Greater Than 0?(x=w447) -> (x > 0?=w452:bool)
                n150 = case shown="True" w452 {
                  tunnel: w451 -> [_ w468]
                  tunnel: w447 -> [_ w467]
                  tunnel: w440 -> [_ w464]
                  tunnel: [FALSE w462] -> w450
                  tunnel: w449 -> [_ w461]
                  tunnel: [u32 0 ("PlanTime (ms)") w457] -> w448
                  frame False {
                  }
                  frame True {
                    n151 = Decrement(x=w467) -> (x-1=w466:i32)
                    n152 = Unbundle By Name(w461) -> ("ArmPlanRequestNotifier"=w460:refnum<notifier>, "ArmPlanResponseNotifier"=w458:refnum<notifier>)
                    n153 = Index Array(array=w468, index=w466) -> (element=w465:T3)
                    n154 = Unbundle By Name(w464) -> ("ArmPosition"=w459:T6)
                    n155 = Unbundle By Name(w465) -> ("ArmPosition"=w463:T6)
                    n156 = Not Equal?(x=w459, y=w463) -> (x != y?=w462:bool)
                    n157 = case shown="True" w462 {
                      tunnel: w460 -> [_ w478]
                      tunnel: w459 -> [_ w475]
                      tunnel: w458 -> [_ w473]
                      tunnel: [u32 0 ("PlanTime (ms)") w470] -> w457
                      frame False {
                      }
                      frame True {
                        n158 = Bundle By Name(cluster=T11 {"Destination"=enum."Hold", "Preview"=FALSE} ("notification"), "Destination"=w475, "Preview"=FALSE) -> (w477:T11)
                        n159 = Send Notification(notification=w477, notifier=w478) -> ()  [unwired: 1 in, 2 out]
                        n160 = Wait on Notification(notifier=w473, ignore previous (F)=TRUE) -> (notification=w471:T8)  [unwired: 2 in, 3 out]
                        n161 = Unbundle By Name(w471) -> ("PlanTime (ms)"=w470:u32)
                      }
                    }
                  }
                }
                n162 = Unbundle By Name(w440) -> ("IntakeState"=w439:T2, "ClawReleaseTime (ms)"=w444:u16, "Claw Open"=w442:bool)
                n163 = Equal To 0?(x=w444) -> (x = 0?=w441:bool)
                n164 = Not(x=w442) -> (.not. x?=w443:bool)
                n165 = Select(t=w442, s=w441, f=w443) -> (s? t:f=w438:bool)
              }
              frame "Vision Assist Endpoint" {
                # "Not implemented yet"
                n166 = Increment(x=w488) -> (x+1=w484:i32)
              }
              frame "Stop" {
              }
            }
            n167 = Tick Count (ms)() -> (millisecond timer value=w279:u32)
          }
        }
      }
    }
    "IntakeState" <- w34
    "Claw Open" <- w33
  }
